vi "Skewness and Kurtosis.vi"(10 "Weighting (Sample)":enum16{"Sample", "Population"}(ring), 11 "X":dbl[](array[numeric])) -> (0 "error":i32, 2 "kurtosis":dbl, 3 "skewness":dbl)   [LabVIEW 2020, in "NI_Gmath.lvlib"]
doc: "Computes the skewness and kurtosis of the input sequence <B>X</B>."
uses:
  NI_Gmath.lvlib
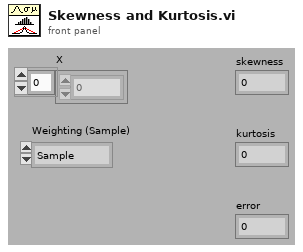
[diagram p1: front panel]
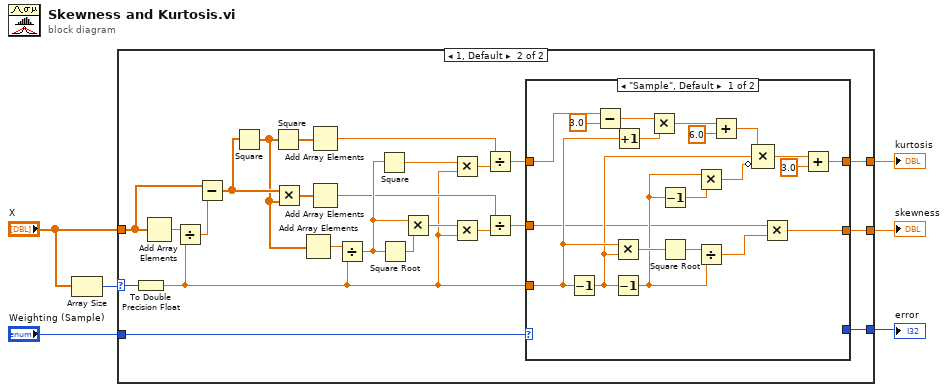
[diagram p0: block diagram]
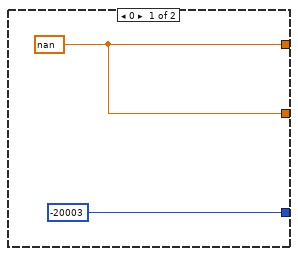
[diagram p2: hidden frame]
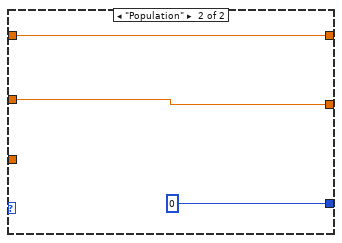
[diagram p3: hidden frame]
diagram:
  n1 = Array Size(array="X") -> (size(s)=w1:i32)
  n2 = case shown="1, Default" w1 {
    selector: w1 -> [_ w9]
    tunnel: "X" -> [_ w32]
    tunnel: "Weighting (Sample)" -> [_ w16]
    tunnel: [w8 w13] -> w4
    tunnel: [w8 w12] -> w3
    tunnel: [-20003 w11] -> w2
    frame 0 {
      w8 = nan
    }
    frame 1, Default {
      n3 = To Double Precision Float(number=w9) -> (double precision float=w10:dbl)
      n4 = Add Array Elements(numeric array=w32) -> (sum=w31:dbl)
      n5 = Divide(x=w31, y=w10) -> (x/y=w30:dbl)
      n6 = Subtract(x=w32, y=w30) -> (x-y=w19:dbl[])
      n7 = Square(x=w19) -> (x^2=w18:dbl[])
      n8 = Square(x=w18) -> (x^2=w17:dbl[])
      n9 = Multiply(x=w19, y=w18) -> (x*y=w28:dbl[])
      n10 = Add Array Elements(numeric array=w18) -> (sum=w29:dbl)
      n11 = Add Array Elements(numeric array=w17) -> (sum=w23:dbl)
      n12 = Add Array Elements(numeric array=w28) -> (sum=w21:dbl)
      n13 = Divide(x=w29, y=w10) -> (x/y=w26:dbl)
      n14 = Square(x=w26) -> (x^2=w24:dbl)
      n15 = Square Root(x=w26) -> (sqrt(x)=w27:dbl)
      n16 = Multiply(x=w26, y=w27) -> (x*y=w25:dbl)
      n17 = Multiply(x=w24, y=w10) -> (x*y=w22:dbl)
      n18 = Multiply(x=w25, y=w10) -> (x*y=w20:dbl)
      n19 = Divide(x=w23, y=w22) -> (x/y=w15:dbl)
      n20 = Divide(x=w21, y=w20) -> (x/y=w14:dbl)
      n21 = case shown="\"Sample\", Default" w16 {
        tunnel: w15 -> [w42 w55]
        tunnel: w14 -> [w33 w54]
        tunnel: [w41 w55] -> w13
        tunnel: [w40 w54] -> w12
        tunnel: [_ 0] -> w11
        tunnel: w10 -> [w39 _]
        frame "Sample", Default {
          n22 = Decrement(x=w39) -> (x-1=w38:dbl)
          n23 = Subtract(x=w42, y=3.0) -> (x-y=w48:dbl)
          n24 = Multiply(x=w39, y=w38) -> (x*y=w52:dbl)
          n25 = Decrement(x=w38) -> (x-1=w34:dbl)
          n26 = Increment(x=w39) -> (x+1=w47:dbl)
          n27 = Multiply(x=w48, y=w47) -> (x*y=w46:dbl)
          n28 = Decrement(x=w34) -> (x-1=w35:dbl)
          n29 = Square Root(x=w52) -> (sqrt(x)=w51:dbl)
          n30 = Multiply(x=w34, y=w35) -> (x*y=w36:dbl)
          n31 = Divide(x=w51, y=w34) -> (x/y=w50:dbl)
          n32 = Add(x=w46, y=6.0) -> (x+y=w37:dbl)
          n33 = Compound Arithmetic op=MULTIPLY(w37, w38, invert w36) -> (w44:dbl)
          n34 = Multiply(x=w33, y=w50) -> (x*y=w40:dbl)
          n35 = Add(x=w44, y=3.0) -> (x+y=w41:dbl)
        }
        frame "Population" {
        }
      }
    }
  }
  "skewness" <- w3
  "kurtosis" <- w4
  "error" <- w2
